vi "AdjustSpeaker_old.vi"(5 "Peiker_Stepped Sweep Settings":T2={"Input Settings"={"IEPE min time to settle [s]"=0.0, "Responce Channel Settings"={"DSA response channel settings"={"coupling"=10045, "enable IEPE excitation"=FALSE, "IEPE current [mA]"=4.0}, "response channel info"={"sensor sensitivity [mV/EU]"=200.0, "engineering units"=2, "dB reference [EU]"=2e-05, "custom label"="EU", "weighting filter"=0, "pregain [dB]"=0.0}, "AI response settings"={"response channel"="SOUNDACQ/ai1", "max value [V]"=10.0, "min value [V]"=-10.0, "terminal configuration"=-1}}, "Stimulus Channel Settings"={"AI stimulus settings"={"stimulus channel"="SOUNDACQ/ai0", "max value [V]"=10.0, "min value [V]"=-10.0, "terminal configuration"=-1}, "DSA stimulus channel settings"={"coupling"=10045, "enable IEPE excitation"=TRUE, "IEPE current [mA]"=4.0}, "stimulus channel info"={"sensor sensitivity [mV/EU]"=11.4, "engineering units"=2, "dB reference [EU]"=2e-05, "custom label"="EU", "weighting filter"=0, "pregain [dB]"=0.0}}}, "Output Settings"={"AO source settings"={"excitation channel"="SOUNDACQ/ao0", "max value [V]"=10.0, "min value [V]"=-10.0, "terminal configuration"=-1}}} {"Output Settings"."AO source settings"."terminal configuration" items=["Default"=-1, "RSE"=10083, "Differential"=10106, "Pseudodifferential"=12529]; "Output Settings"."AO source settings"."min value [V]" format="%0.2f"; "Output Settings"."AO source settings"."max value [V]" format="%0.2f"; "Input Settings"."Stimulus Channel Settings"."stimulus channel info"."pregain [dB]" format="%.2f"; "Input Settings"."Stimulus Channel Settings"."stimulus channel info"."weighting filter" items=["Linear", "A-weighting", "B-weighting", "C-weighting", "ITU-R 468-4", "Dolby", "CCITT", "C-message", "Wb", "Wc", "Wd", "We", "Wf", "Wh", "Wj", "Wk", "Wm", "AES17 20 kHz lowpass", "AES17 40 kHz lowpass", "AES17 20 kHz highpass", "AES17 40 kHz highpass"]; "Input Settings"."Stimulus Channel Settings"."stimulus channel info"."dB reference [EU]" format="%^.1e"; "Input Settings"."Stimulus Channel Settings"."stimulus channel info"."engineering units" items=["custom..."=0, "V"=1, "A"=21, "Pa"=2, "N"=20, "g"=3, "m/s^2"=4, "m/s"=5, "m"=6, "mm/s"=12, "mm"=13, "micron/s"=14, "micron"=15, "in/s^2"=7, "in/s"=8, "in"=9, "mil/s"=10, "mil"=11, "rad/s^2"=16, "rad/s"=17, "rad"=18, "deg/s^2"=26, "deg/s"=27, "deg"=28, "RPM"=22, "cycle/s^2"=23, "Hz"=24, "cycle"=25, "strain"=19]; "Input Settings"."Stimulus Channel Settings"."stimulus channel info"."sensor sensitivity [mV/EU]" format="%.2f"; "Input Settings"."Stimulus Channel Settings"."DSA stimulus channel settings"."IEPE current [mA]" format="%.1f"; "Input Settings"."Stimulus Channel Settings"."DSA stimulus channel settings"."coupling" items=["AC"=10045, "DC"=10050, "GND"=10066]; "Input Settings"."Stimulus Channel Settings"."AI stimulus settings"."terminal configuration" items=["Default"=-1, "RSE"=10083, "NRSE"=10078, "Differential"=10106, "Pseudodifferential"=12529]; "Input Settings"."Stimulus Channel Settings"."AI stimulus settings"."min value [V]" format="%.2f"; "Input Settings"."Stimulus Channel Settings"."AI stimulus settings"."max value [V]" format="%.2f"; "Input Settings"."Responce Channel Settings"."AI response settings"."terminal configuration" items=["Default"=-1, "RSE"=10083, "NRSE"=10078, "Differential"=10106, "Pseudodifferential"=12529]; "Input Settings"."Responce Channel Settings"."AI response settings"."min value [V]" format="%.2f"; "Input Settings"."Responce Channel Settings"."AI response settings"."max value [V]" format="%.2f"; "Input Settings"."Responce Channel Settings"."response channel info"."pregain [dB]" format="%.2f"; "Input Settings"."Responce Channel Settings"."response channel info"."weighting filter" items=["Linear", "A-weighting", "B-weighting", "C-weighting", "ITU-R 468-4", "Dolby", "CCITT", "C-message", "Wb", "Wc", "Wd", "We", "Wf", "Wh", "Wj", "Wk", "Wm", "AES17 20 kHz lowpass", "AES17 40 kHz lowpass", "AES17 20 kHz highpass", "AES17 40 kHz highpass"]; "Input Settings"."Responce Channel Settings"."response channel info"."dB reference [EU]" format="%^.1e"; "Input Settings"."Responce Channel Settings"."response channel info"."engineering units" items=["custom..."=0, "V"=1, "A"=21, "Pa"=2, "N"=20, "g"=3, "m/s^2"=4, "m/s"=5, "m"=6, "mm/s"=12, "mm"=13, "micron/s"=14, "micron"=15, "in/s^2"=7, "in/s"=8, "in"=9, "mil/s"=10, "mil"=11, "rad/s^2"=16, "rad/s"=17, "rad"=18, "deg/s^2"=26, "deg/s"=27, "deg"=28, "RPM"=22, "cycle/s^2"=23, "Hz"=24, "cycle"=25, "strain"=19]; "Input Settings"."Responce Channel Settings"."response channel info"."sensor sensitivity [mV/EU]" format="%.2f"; "Input Settings"."Responce Channel Settings"."DSA response channel settings"."IEPE current [mA]" format="%.1f"; "Input Settings"."Responce Channel Settings"."DSA response channel settings"."coupling" items=["AC"=10045, "DC"=10050, "GND"=10066]; "Input Settings"."IEPE min time to settle [s]" format="%.1f"}, 7 "SollPegel/dBSPL":i32=94, 8 "error in":errorcluster, 9 "integration time":T9={"integration time [s]"=0.015599999576807022, "integration cycles"=5} {"integration cycles" min=2; "integration time [s]" format="%.2p"}, 10 "settling time":T8={"settle time [s]"=0.015599999576807022, "settle cycles"=5} {"settle time [s]" format="%.2p"}, 11 "Frequency List":T1(array[cluster])) -> (0 "error out":errorcluster, 2 "magnitude":dbl[](array[numeric]), 3 "korrigierte Frequenzliste":T1(array[cluster]))   [LabVIEW 2012]
uses:
  Peiker_Stepped Sweep Settings.ctl
  <vilib>/addons/_NISVFA/_Shared subVIs/Controls/svc_DSA Channel Settings.ctl
  <vilib>/addons/_NISVFA/_Shared subVIs/Controls/svc_Channel Info.ctl
  <vilib>/addons/_NISVFA/_Shared subVIs/Controls/svc_Engineering Units Text Ring.ctl
  <vilib>/addons/_NISVFA/_Shared subVIs/Controls/svc_Weighting Filter Text Ring.ctl
panel:
  out "Array":dbl[][](array[numeric])
  out "magnitude 2":dbl[][](array[numeric])
  out "Durchläufe":i32
  out "alle Frequenzlisten":T7(array[cluster])
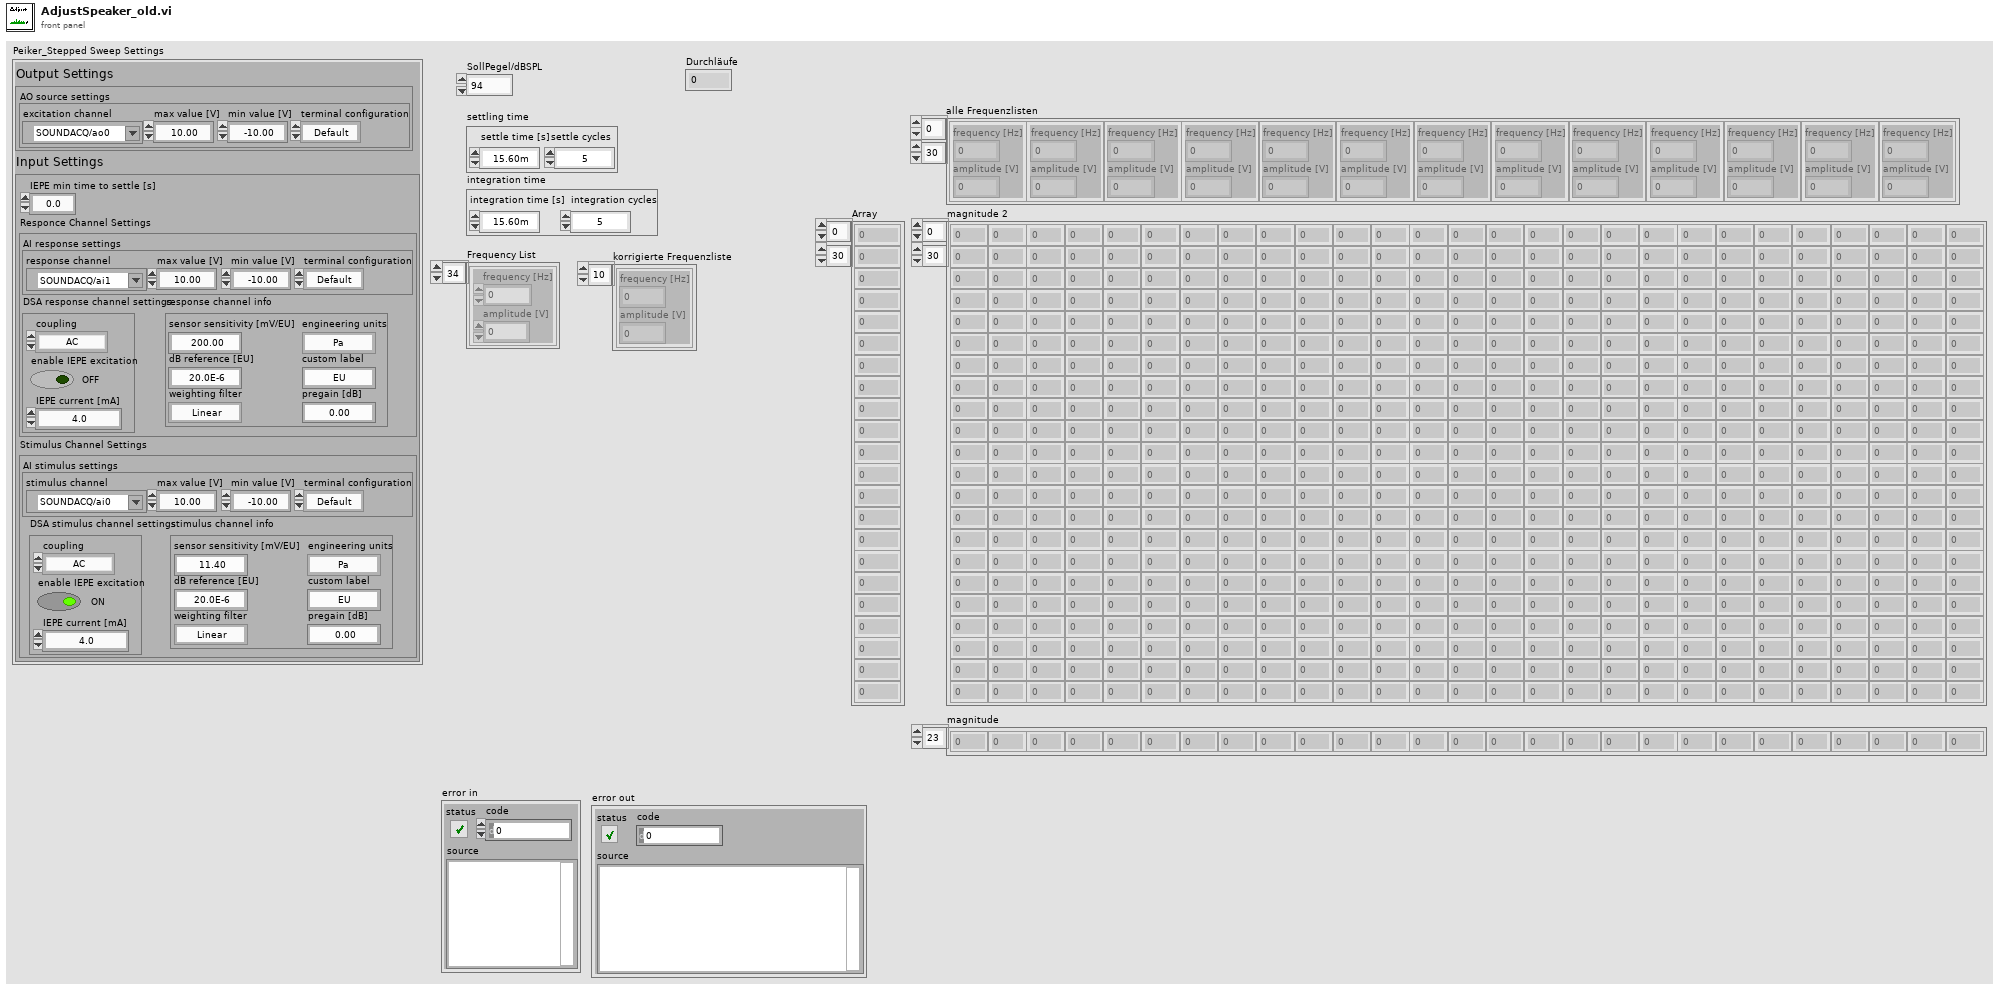
[diagram p1: front panel]
types:
  T1 = cluster{"frequency [Hz]":dbl, "amplitude [V]":dbl}[]
  T2 = typedef "Peiker_Stepped Sweep Settings.ctl" = cluster{"Input Settings":cluster{"IEPE min time to settle [s]":dbl, "Responce Channel Settings":cluster{"DSA response channel settings":T3, "response channel info":T4, "AI response settings":cluster{"response channel":tag, "max value [V]":dbl, "min value [V]":dbl, "terminal configuration":i32}}, "Stimulus Channel Settings":cluster{"AI stimulus settings":cluster{"stimulus channel":tag, "max value [V]":dbl, "min value [V]":dbl, "terminal configuration":i32}, "DSA stimulus channel settings":T3, "stimulus channel info":T4}}, "Output Settings":cluster{"AO source settings":cluster{"excitation channel":tag, "max value [V]":dbl, "min value [V]":dbl, "terminal configuration":i32}}}
  T3 = typedef "svc_DSA Channel Settings.ctl" = cluster{"coupling":i32, "enable IEPE excitation":bool, "IEPE current [mA]":dbl}
  T4 = typedef "svc_Channel Info.ctl" = cluster{"sensor sensitivity [mV/EU]":dbl, "engineering units":T5, "dB reference [EU]":dbl, "custom label":string, "weighting filter":T6, "pregain [dB]":dbl}
  T5 = typedef "svc_Engineering Units Text Ring.ctl" = u16
  T6 = typedef "svc_Weighting Filter Text Ring.ctl" = u16
  T7 = cluster{"frequency [Hz]":dbl, "amplitude [V]":dbl}[][]
  T8 = cluster{"settle time [s]":dbl, "settle cycles":i32}
  T9 = cluster{"integration time [s]":dbl, "integration cycles":i32}
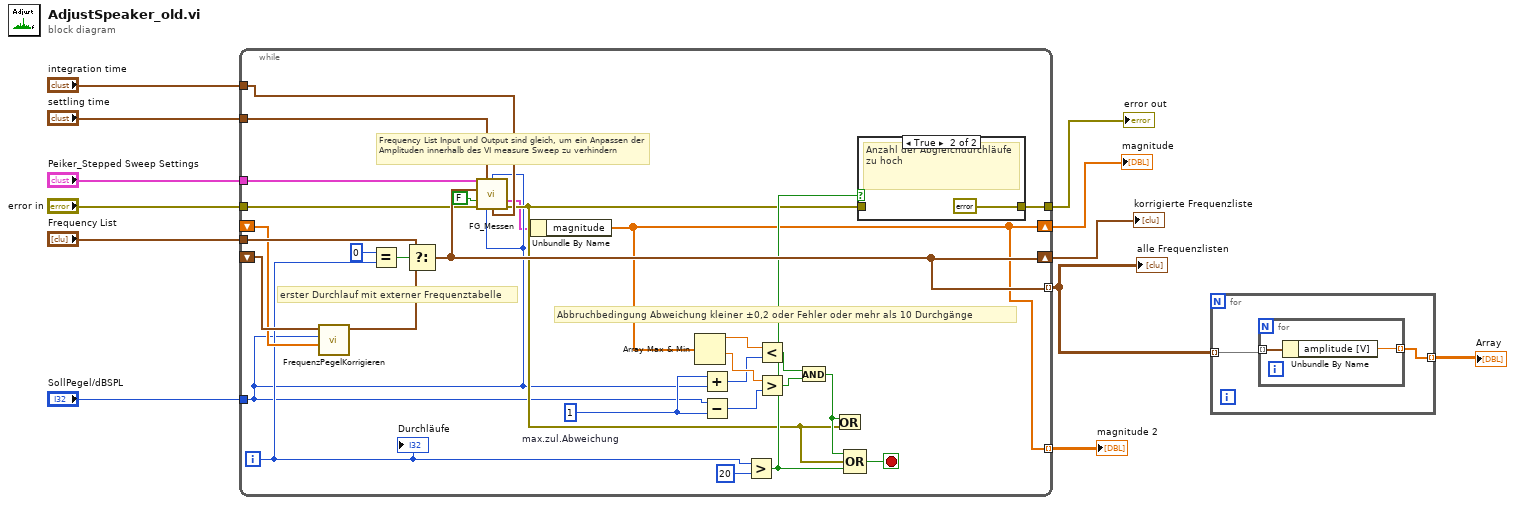
[diagram p0: block diagram]
diagram:
  n1 = while {
    tunnel: "Peiker_Stepped Sweep Settings" -> [w27]
    tunnel: "Frequency List" -> [w32]
    shift-right: [w28] -> w10
    shift-left: _ -> [w30]
    shift-right: [w14] -> w4
    shift-left: _ -> [w29]
    tunnel: [w28] -> w2 mode=indexing
    tunnel: "error in" -> [w26]
    tunnel: "integration time" -> [w24]
    tunnel: "settling time" -> [w23]
    tunnel: "SollPegel/dBSPL" -> [w15]
    tunnel: [w16] -> w5
    tunnel: [w14] -> w3 mode=indexing
    i -> [w21]
    stop <- w19 stop-if-true
    w35 = 1  # max.zul.Abweichung
    # "Frequency List Input und Output sind gleich, um ein Anpassen der Amplituden innerhalb des VI measure Sweep zu verhindern"
    # "erster Durchlauf mit externer Frequenztabelle"
    # "Abbruchbedingung Abweichung kleiner ±0,2 oder Fehler oder mehr als 10 Durchgänge"
    n2 = call "FrequenzPegelKorrigieren.vi"("gemessenerPegel"=w29, "SollPegel"=w15, "Frequency List"=w30) -> ("korrigierte Frequenzliste"=w31:T1)  [unwired: 8 in]
    n3 = Equal?(x=0, y=w21) -> (x = y?=w33:bool)
    n4 = Select(t=w32, s=w33, f=w31) -> (s? t:f=w28:T1)
    n5 = call "FG_Messen.vi"("Peiker_Stepped Sweep Settings"=w27, "settling time"=w23, "FrequencyList Output Level (dBSPL)"=w15, "frequency list Input"=w28, "true=mehrfach Messen"=FALSE, "error in (no error)"=w26, "FrequencyList Input Level (dBSPL)"=w15, "integration time"=w24) -> ("Response Level"=w13:cluster{"frequency":dbl[], "magnitude":dbl[]}, "error out"=w17:errorcluster)  [unwired: 2 in, 4 out]
    n6 = Unbundle By Name(w13) -> ("magnitude"=w14:dbl[])
    n7 = Array Max & Min(array=w14) -> (max value=w41:dbl, min value=w38:dbl)  [unwired: 2 out]
    n8 = Add(x=w35, y=w15) -> (x+y=w37:i32)
    n9 = Subtract(x=w15, y=w35) -> (x-y=w36:i32)
    n10 = Greater?(x=w21, y=20) -> (0:w18:bool)
    n11 = Less?(x=w41, y=w37) -> (x < y?=w40:bool)
    n12 = Greater?(x=w38, y=w36) -> (0:w39:bool)
    n13 = And(x=w40, y=w39) -> (x .and. y?=w22:bool)
    n14 = Or(x=w22, y=w17) -> ()  [unwired: 1 out]
    n15 = Compound Arithmetic op=OR(w22, w17, w18) -> (w19:bool)
    n16 = case shown="True" w18 {
      tunnel: w17 -> [w42 _]
      tunnel: [w42 errorcluster {"status"=TRUE, "code"=5000, "source"="Anzahl der Abgleichdurchgänge zu hoch,\nPrüfen ob der Messaufbau korrekt ist."} ("error out 2")] -> w16
      frame False {
      }
      frame True {
        # "Anzahl der Abgleichdurchläufe zu hoch"
      }
    }
    "Durchläufe" <- w21
  }
  "alle Frequenzlisten" <- w2
  "error out" <- w5
  "korrigierte Frequenzliste" <- w10
  "magnitude" <- w4
  "magnitude 2" <- w3
  n17 = for {
    tunnel: w2 -> [w45] mode=indexing
    tunnel: [w44] -> w1 mode=indexing
    n18 = for {
      tunnel: w45 -> [w47] mode=indexing
      tunnel: [w46] -> w44 mode=indexing
      n19 = Unbundle By Name(w47) -> ("amplitude [V]"=w46:dbl)
    }
  }
  "Array" <- w1
